vi "Aux CO2 Prompt For Zero.vi"(8 "error in":errorcluster, 9 "sequence in":i64[](array[numeric]), 10 "AuxCO2info":T2={"Port"="", "Source"=0, "Active"=FALSE, "Baro Pressure"=760, "SerialRxBuffer"="", "Raw CO2 (Torr)"=5.0, "bytes read"=5, "Status"=[], "Status Message"=enum.""} {"Status" format="%x"; "Baro Pressure" min=400 max=800; "Source" items=["None", "TidalWave", "LoFlow / Canary", "Capnogard"]}, 11 "AuxCO2Port":T4={"termination char"=10, "End read on termination character?"=TRUE, "Enabled?"=TRUE, "VISA resource name"="COM1", "baud rate"=9600, "data bits"=8, "parity"=enum."None", "stop bits"=10, "flow control"=0, "timeout (ms)"=10000, "Input buffer size"=4096, "End write on termination character?"=FALSE, "XON Char"=17, "XOFF Char"=19} {"XOFF Char" format="%.0x"; "XON Char" format="%.0x"; "flow control" items=["None"=0, "XON/XOFF"=1, "RTS/CTS"=2, "DTR/DSR"=4]; "stop bits" items=["1.0"=10, "1.5"=15, "2.0"=20]; "baud rate" items=["1.0"=10, "1.5"=15, "2.0"=20]; "termination char" format="%.0x"}) -> (0 "error out":errorcluster, 1 "sequence out":i64[](array[numeric]), 2 "AuxCO2info out":T2={"Port"="", "Source"=0, "Active"=FALSE, "Baro Pressure"=760, "SerialRxBuffer"="", "Raw CO2 (Torr)"=5.0, "bytes read"=5, "Status"=[], "Status Message"=enum.""} {"Status" format="%x"; "Baro Pressure" min=400 max=800; "Source" items=["None", "TidalWave", "LoFlow / Canary", "Capnogard"]}, 3 "AuxCO2Port out":T4={"termination char"=10, "End read on termination character?"=TRUE, "Enabled?"=TRUE, "VISA resource name"="COM1", "baud rate"=9600, "data bits"=8, "parity"=enum."None", "stop bits"=10, "flow control"=0, "timeout (ms)"=10000, "Input buffer size"=4096, "End write on termination character?"=FALSE, "XON Char"=17, "XOFF Char"=19} {"XOFF Char" format="%.0x"; "XON Char" format="%.0x"; "flow control" items=["None"=0, "XON/XOFF"=1, "RTS/CTS"=2, "DTR/DSR"=4]; "stop bits" items=["1.0"=10, "1.5"=15, "2.0"=20]; "baud rate" items=["1.0"=10, "1.5"=15, "2.0"=20]; "termination char" format="%.0x"})   [LabVIEW 2016]
doc: "sldafkhasdhf;oihdsoifa"
uses:
  Controls/Serial Visa Control.ctl
  Controls/Aux CO2 Diags.ctl
  Controls/Aux CO2 Selector.ctl
  Controls/SerialPortControl.ctl
panel:
  out "Zero In Process":bool
  out "Zero Required":bool
  out "Zero Status":T1(ring)
  out "CO2 Errors":string[](array[string])
  out "Baro Pressure":u16
  out "CO2 (%)":sgl format="%.2f"
  out "CO2 (Torr)":sgl
  out "Status Message":T5(ring)
  out "Status":u8[](array[numeric]) format="%x"
  out "Port Active":bool
  in  "Zero Cmd":bool
  in  "Stop Button":bool
  out "Waveform Chart":sgl(graph)
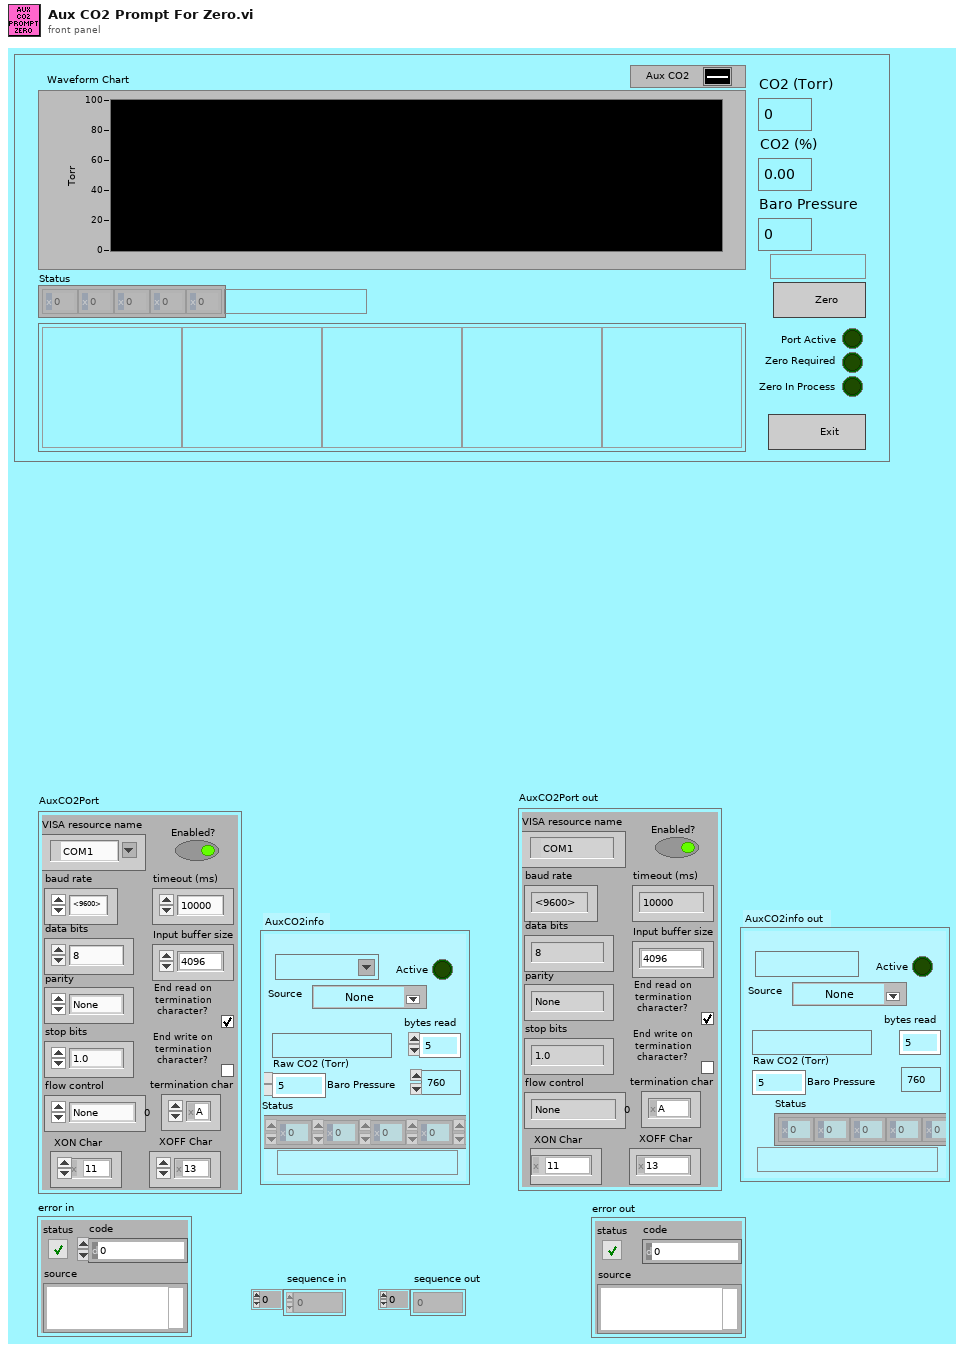
[diagram p1: front panel]
types:
  T1 = enum16{" ", "Zero In Progress", "Zero Required", "Zero Error"}
  T2 = typedef "Aux CO2 Diags.ctl" = cluster{"Port":refnum<visa-resource-name>, "Source":T3, "Active":bool, "Baro Pressure":u16, "SerialRxBuffer":string, "Raw CO2 (Torr)":sgl, "bytes read":i16, "Status":u8[], "Status Message":enum16{"", "Sensor Over Temp", "Sensor Faulty", "Set BaroP", "Capno in Sleep Mode", "Zero In Progress", "Sensor Warm Up", "Check Sampling Line", "Zero Required", "CO2 Out Of Range", "Check Airway Adapter", "LoFlo Not Connected"}}
  T3 = typedef "Aux CO2 Selector.ctl" = u16
  T4 = typedef "Serial Visa Control.ctl" = cluster{"termination char":u8, "End read on termination character?":bool, "Enabled?":bool, "VISA resource name":refnum<visa-resource-name>, "baud rate":u32, "data bits":u16, "parity":enum16{"None", "Odd", "Even", "Mark", "Space"}, "stop bits":u16, "flow control":u16, "timeout (ms)":u32, "Input buffer size":u32, "End write on termination character?":bool, "XON Char":u8, "XOFF Char":u8}
  T5 = enum16{"", "Sensor Over Temp", "Sensor Faulty", "Set BaroP", "Capno in Sleep Mode", "Zero In Progress", "Sensor Warm Up", "Check Sampling Line", "Zero Required", "CO2 Out Of Range", "Check Airway Adapter", "LoFlo Not Connected"}
  T6 = typedef "SerialPortControl.ctl" = enum16{"Initialize", "Write Data", "Read Data", "Close Port"}
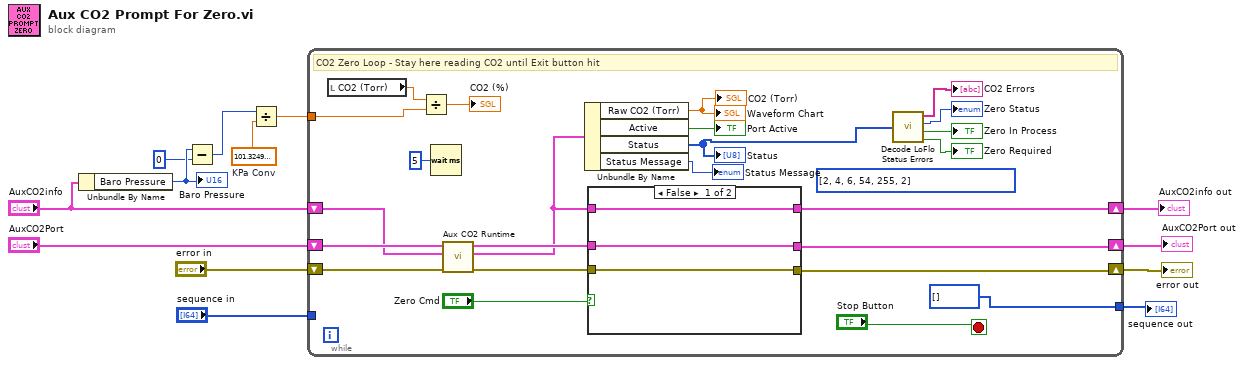
[diagram p0: block diagram]
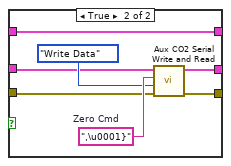
[diagram p2: hidden frame]
diagram:
  w4 = sgl 101.325  # KPa Conv
  n1 = Unbundle By Name("AuxCO2info") -> ("Baro Pressure"=w2:u16)
  "Baro Pressure" <- w2
  n2 = Subtract(x=w2, y=u16 0) -> (x-y=w5:u16)
  n3 = Divide(x=w5, y=w4) -> (x/y=w3:sgl)
  n4 = while {
    shift-right: [w25] -> w8
    shift-left: "AuxCO2info" -> [w34]
    shift-right: [w28] -> w7
    shift-left: "AuxCO2Port" -> [w36]
    shift-right: [w27] -> w11
    shift-left: "error in" -> [w35]
    tunnel: "sequence in" -> [_]
    tunnel: [i64[] [] ("sequence out")] -> w9
    tunnel: w3 -> [w21]
    stop <- "Stop Button" stop-if-true
    (unwired) u8[] [2, 4, 6, 54, 255, 2] ("Status")
    # "CO2 Zero Loop - Stay here reading CO2 until Exit button hit"
    n5 = local read "CO2 (Torr)"() -> (w20:sgl)
    n6 = Divide(x=w20, y=w21) -> (x/y=→"CO2 (%)":sgl)
    n7 = Wait (ms)(milliseconds to wait=u32 5) -> ()  [unwired: 1 out]
    n8 = call "Aux CO2 Runtime.vi"("Error In"=w35, "Capno Data In"=w34, "Serial Port In"=w36) -> ("Error Out"=w30:errorcluster, "Capno Data Out"=w26:T2, "Serial Port Out"=w31:T4)  [unwired: 5 in, 1 out]
    n9 = Unbundle By Name(w26) -> ("Raw CO2 (Torr)"=→"Waveform Chart" →"CO2 (Torr)":sgl, "Active"=→"Port Active":bool, "Status"=w14:u8[], "Status Message"=→"Status Message":T5)
    "Status" <- w14
    n10 = case shown="False" "Zero Cmd" {
      tunnel: w31 -> [w39 w45]
      tunnel: w30 -> [w38 w44]
      tunnel: [w39 w43] -> w28
      tunnel: [w38 w42] -> w27
      tunnel: [w40 w41] -> w25
      tunnel: w26 -> [w40 w41]
      frame False {
      }
      frame True {
        w47 = "‚\u0001}"  # Zero Cmd
        n11 = call "Aux CO2 Serial Write and Read.vi"("error in"=w44, "Action"=SerialPortControl."Write Data", "string to write"=w47, "Serial Port"=w45) -> ("error IO"=w42:errorcluster, "Serial Port Out"=w43:T4)  [unwired: 2 out]
      }
    }
    n12 = call "Decode LoFlo Status Errors.vi"("Status"=w14) -> ("CO2 Errors"=→"CO2 Errors":string[], "Zero Status"=→"Zero Status":T1, "Zero In Process"=→"Zero In Process":bool, "Zero Required"=→"Zero Required":bool)
  }
  "sequence out" <- w9
  "error out" <- w11
  "AuxCO2Port out" <- w7
  "AuxCO2info out" <- w8
